vi "总磷插入数据.vi"(0 "database":string, 1 "data":T1 {"单位" items=["ug/L", "mg/L", "ppm", "mg/m3", "cm", "ppb", "ug/m3", "%", "nmol/mol", "umol/mol", "MPN/L", "MPN/100ml", "ng/m3", "NTU", "无量纲", "ms/cm", "us/cm"]}, 3 "SN":string, 5 "table":string, 7 "测量模式":T2(ring)=enum."水样测试", 9 "数据标记表":string(combo)="N", 11 "error in (no error)":errorcluster) -> (15 "error out":errorcluster)   [LabVIEW 2016, in "斯坦道总氮.lvlib"]
uses:
  <vilib>/Utility/sysdir.llb/System Directory Type.ctl
  <vilib>/addons/database/Connection.llb/DB Tools Open Connec (String).vi
  <vilib>/addons/database/Connection.llb/Conn Execute.vi
  <vilib>/addons/database/Recordset.llb/Rec Destroy - Connection.vi
  <vilib>/addons/database/Recordset.llb/Rec Fetch Recordset Data (R).vi
  <vilib>/addons/database/NI_Database_API.lvlib
panel:
  out "为空？":bool
  out "recordset data":variant[][](array[variant])
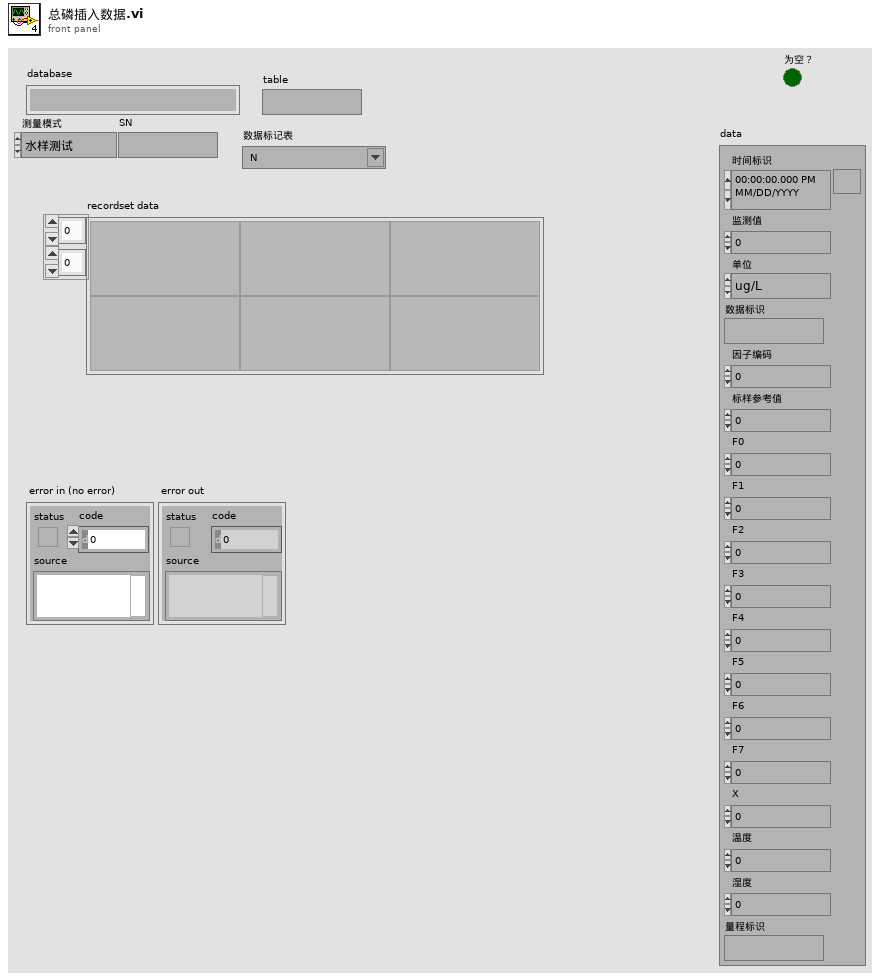
[diagram p1: front panel]
types:
  T1 = cluster{"时间标识":timestamp, "监测值":sgl, "单位":u16, "数据标识":string, "因子编码":u32, "标样参考值":sgl, "F0":sgl, "F1":sgl, "F2":sgl, "F3":sgl, "F4":sgl, "F5":sgl, "F6":sgl, "F7":sgl, "X":sgl, "温度":sgl, "湿度":sgl, "量程标识":string}
  T2 = enum16{"维护数据", "水样测试", "标样核查", "零点核查", "跨度核查", "空白测试", "平行样测试", "加标回收", "空白校准", "标样校准", "初始化（清洗）"}
  T3 = typedef "System Directory Type.ctl" = i32
  T4 = typedef "NI_Database_API.lvlib/Conn ObjectReference.ctl" = refnum<k1>
  T5 = typedef "NI_Database_API.lvlib/Rec ObjectReference.ctl" = refnum<k1>
  T6 = cluster{"时间标识":timestamp, "测量模式":string, "数据类型":string, "监测值":sgl, "单位":string, "数据标识":string, "因子编码":string, "标样参考值":sgl, "F0":sgl, "F1":sgl, "F2":sgl, "F3":sgl, "F4":sgl, "F5":sgl, "F6":sgl, "F7":sgl, "X":sgl, "温度":sgl, "湿度":sgl, "量程标识":string, "SN":string, "Last Time":timestamp}
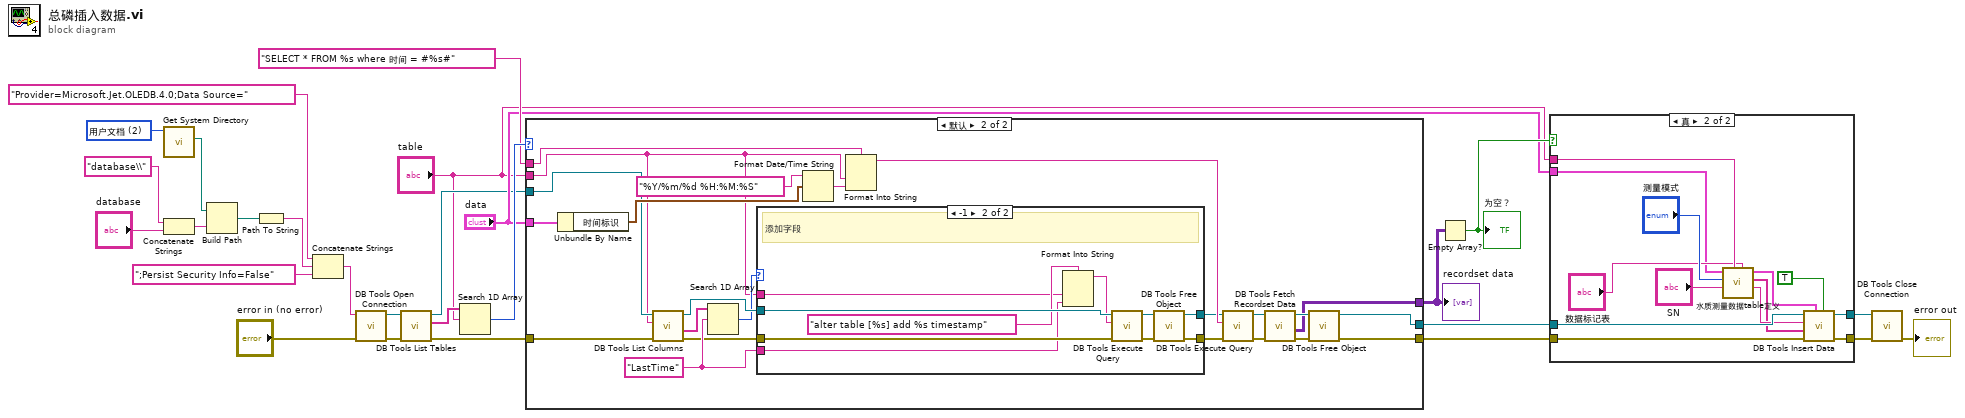
[diagram p0: block diagram]
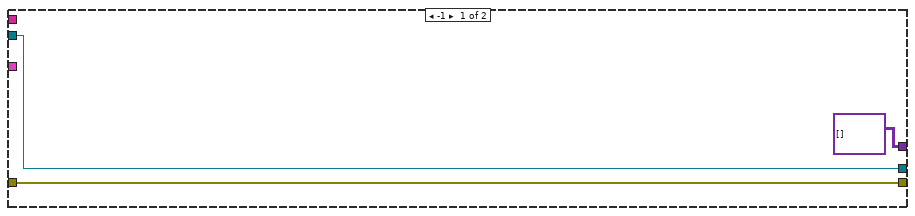
[diagram p3: hidden frame]
diagram:
  w26 = T3 2 items=["用户目录"=0, "用户桌面"=1, "用户文档"=2, "用户应用程序数据"=3, "用户设置"=4, "用户临时目录"=5, "公共文档"=6, "公共应用程序数据"=7, "公共设置"=8, "公共缓存"=13, "系统核心库"=9, "系统安装库"=10, "应用程序文件"=11, "启动盘根目录"=12] ("system directory type")
  n1 = call <vilib>:"Get System Directory.vi"("system directory type"=w26) -> ("system directory"=w24:path)  [unwired: 10 in]
  n2 = Concatenate Strings("database\\" ("condition"), "database") -> (w18:string)
  n3 = Build Path(base path=w24, name or relative path=w18) -> (appended path=w23:path)
  n4 = Path To String(path=w23) -> (string=w22:string)
  n5 = Concatenate Strings("Provider=Microsoft.Jet.OLEDB.4.0;Data Source=" ("condition"), w22, ";Persist Security Info=False" ("condition")) -> (w20:string)
  n6 = call-poly <vilib>:"DB Tools Open Connection.vi"("error in (no error)"="error in (no error)", "connection information"=w20) -> ("error out"=w15:errorcluster, "connection reference"=w16:T4)  [unwired: 6 in]
  n7 = call <vilib>:"DB Tools List Tables.vi"("error in (no error)"=w15, "connection reference"=w16) -> ("error out"=w2:errorcluster, "tables"=w14:string[], "connection reference out"=w3:T4)  [unwired: 3 in]
  n8 = Search 1D Array(1D array=w14, element="table") -> (index of element=w13:i32)  [unwired: 1 in]
  n9 = case shown="默认" w13 {
    tunnel: [variant[][] [] ("recordset data") w49] -> w17
    tunnel: [w30 w48] -> w8
    tunnel: [w29 w47] -> w9
    tunnel: w3 -> [w30 w33]
    tunnel: w2 -> [w29 w32]
    tunnel: "table" -> [_ w31]
    tunnel: "SELECT * FROM %s where 时间 = #%s#" ("格式字符串") -> [_ w46]
    tunnel: "data" -> [_ w41]
    frame -1 {
    }
    frame Default {
      w39 = "LastTime" ("元素")
      n10 = Unbundle By Name(w41) -> ("时间标识"=w44:timestamp)
      n11 = call <vilib>:"DB Tools List Columns.vi"("error in (no error)"=w32, "table"=w31, "connection reference"=w33) -> ("error out"=w37:errorcluster, "columns"=w38:string[], "connection reference out"=w40:T4)  [unwired: 1 in, 1 out]
      n12 = Search 1D Array(1D array=w38, element=w39) -> (index of element=w36:i32)  [unwired: 1 in]
      n13 = case shown="-1" w36 {
        tunnel: w40 -> [w55 w63]
        tunnel: w37 -> [w54 w62]
        tunnel: w39 -> [_ w60]
        tunnel: [w55 w58] -> w35
        tunnel: [w54 w57] -> w34
        tunnel: w31 -> [_ w56]
        frame 0, Default {
        }
        frame -1 {
          # "添加字段"
          n14 = Format Into String(format string="alter table [%s] add %s timestamp", w56, w60) -> (resulting string=w59:string)  [unwired: 2 in, 1 out]
          n15 = call-poly <vilib>:"DB Tools Execute Query.vi"("error in (no error)"=w62, "SQL query"=w59, "connection reference"=w63) -> ("error out"=w64:errorcluster, "recordset reference"=w65:T5)  [unwired: 5 in]
          n16 = call-poly <vilib>:"DB Tools Free Object.vi"("error in (no error)"=w64, "recordset reference"=w65) -> ("error out"=w57:errorcluster, "connection reference"=w58:T4)  [unwired: 8 in]
        }
      }
      n17 = Format Date/Time String(time format string (%c)="%Y/%m/%d %H:%M:%S" ("时间格式字符串(%c)"), seconds (now)=w44) -> (date/time string=w42:string)  [unwired: 1 in]
      n18 = Format Into String(format string=w46, w31, w42) -> (resulting string=w45:string)  [unwired: 2 in, 1 out]
      n19 = call-poly <vilib>:"DB Tools Execute Query.vi"("error in (no error)"=w34, "SQL query"=w45, "connection reference"=w35) -> ("error out"=w50:errorcluster, "recordset reference"=w53:T5)  [unwired: 5 in]
      n20 = call-poly <vilib>:"DB Tools Fetch Recordset Data.vi"("error in (no error)"=w50, "recordset reference"=w53) -> ("error out"=w51:errorcluster, "recordset data"=w49:variant[][], "recordset reference out"=w52:T5)  [unwired: 3 in]
      n21 = call-poly <vilib>:"DB Tools Free Object.vi"("error in (no error)"=w51, "recordset reference"=w52) -> ("error out"=w47:errorcluster, "connection reference"=w48:T4)  [unwired: 8 in]
    }
  }
  "recordset data" <- w17
  n22 = Empty Array?(array=w17) -> (empty?=w10:bool)
  "为空？" <- w10
  n23 = case shown="真" w10 {
    tunnel: "table" -> [_ w80]
    tunnel: "data" -> [_ w68]
    tunnel: w9 -> [w66 w78]
    tunnel: w8 -> [w67 w77]
    tunnel: [w67 w72] -> w7
    tunnel: [w66 w71] -> w6
    frame False {
    }
    frame True {
      n24 = call "水质测量数据table定义.vi"("数据标记表"="数据标记表", "table 输入"=w80, "SN"="SN", "测量模式"="测量模式", "data"=w68) -> ("table 输出"=w74:string, "columns"=w73:string[], "data输出"=w76:T6)  [unwired: 4 in]
      n25 = call <vilib>:"DB Tools Insert Data.vi"("create table? (F)"=TRUE, "data"=w76, "error in (no error)"=w78, "columns"=w73, "table"=w74, "connection reference"=w77) -> ("error out"=w71:errorcluster, "connection reference out"=w72:T4)  [unwired: 4 in]
    }
  }
  n26 = call <vilib>:"DB Tools Close Connection.vi"("error in (no error)"=w6, "connection reference"=w7) -> ("error out"=→"error out":errorcluster)  [unwired: 5 in]
